vi "Initialize Master.vi"(8 "error in":errorcluster, 11 "TCP master in":refnum<class "TCP Master.lvclass">) -> (0 "error out":errorcluster, 3 "TCP master out":refnum<class "TCP Master.lvclass">)   [LabVIEW 2021, in "TCP Master.lvclass"]
doc: "Opens a TCP connection to the address and port stored in the class."
uses:
  TCP Master.lvclass
  TCP Master.lvclass/TCP Master.ctl
  Network Protocol.lvclass
  Transmission Data Unit/Transmission Data Unit.lvclass
  D:/my_projects/projects/Algorithms/Labview/21/Modbus_v121c/Network Protocol/Network Master/Network Master.lvclass
  D:/my_projects/projects/Algorithms/Labview/21/Modbus_v121c/Network Protocol/Network Protocol.lvclass
  D:/my_projects/projects/Algorithms/Labview/21/Modbus_v121c/Network Protocol/Network Master/TCP/TCP Master.lvclass
  Network Interface/Network Interface.lvclass
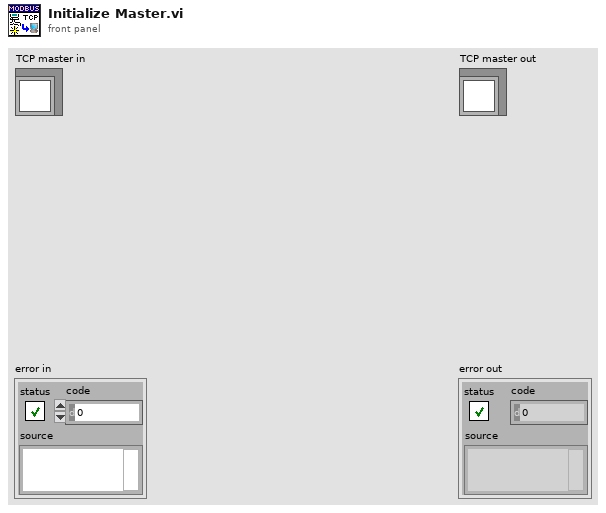
[diagram p1: front panel]
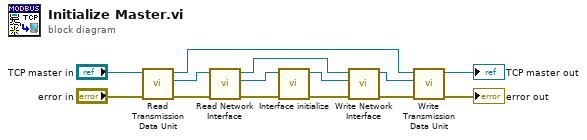
[diagram p0: block diagram]
diagram:
  n1 = call "Read Transmission Data Unit.vi"("error in (no error)"="error in", "Network Protocol in"="TCP master in") -> ("error out"=w8:errorcluster, "Transmission Data Unit"=w13:refnum<class "Transmission Data Unit.lvclass">, "Network Protocol out"=w3:refnum<class "TCP Master.lvclass">)  [unwired: 7 in]
  n2 = call "Read Network Interface.vi"("error in (no error)"=w8, "Transmission Data Unit in"=w13) -> ("error out"=w7:errorcluster, "Network Interface"=w12:refnum<class "Network Interface.lvclass">, "Transmission Data Unit out"=w9:refnum<class "Transmission Data Unit.lvclass">)  [unwired: 7 in]
  n3 = call-dynamic "Interface initialize.vi"("error in"=w7, "interface in"=w12) -> ("error out"=w6:errorcluster, "interface out"=w11:refnum<class "Network Interface.lvclass">)  [unwired: 8 in]
  n4 = call "Write Network Interface.vi"("error in (no error)"=w6, "Network Interface"=w11, "Transmission Data Unit in"=w9) -> ("error out"=w5:errorcluster, "Transmission Data Unit out"=w10:refnum<class "Transmission Data Unit.lvclass">)  [unwired: 7 in]
  n5 = call "Write Transmission Data Unit.vi"("error in (no error)"=w5, "Transmission Data Unit"=w10, "Network Protocol in"=w3) -> ("error out"=→"error out":errorcluster, "Network Protocol out"=→"TCP master out":refnum<class "TCP Master.lvclass">)  [unwired: 7 in]
